vi "Consumer Loop.vi"(8 "error in (no error)":errorcluster) -> (0 "error out":errorcluster)   [LabVIEW 2014]
doc: "Executes the motion commands."
uses:
  Functional_Global/Typedef_Message_Queue_Action.ctl
  Typedef/Typedef_Motor_Message.ctl
  EMC API/EMC_Typedef_Motor_Parameters.ctl
  Typedef/Typedef_Coordinate_Move_Message.ctl
  Globals/Global Stop.vi
panel:
  out "Iterations":i32
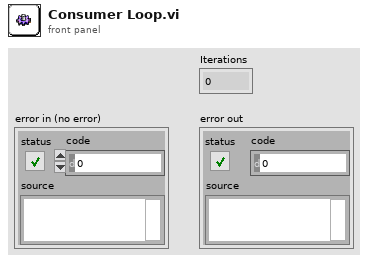
[diagram p1: front panel]
types:
  T1 = typedef "Typedef_Message_Queue_Action.ctl" = enum16{"Init MQueue", "Get MQueue Ref", "Close MQueue"}
  T2 = typedef "Typedef_Motor_Message.ctl" = cluster{"Axis":refnum<k21>, "Motion Parameters":T3}
  T3 = typedef "EMC_Typedef_Motor_Parameters.ctl" = cluster{"position":dbl, "velocity":dbl, "acceleration":dbl, "deceleration":dbl, "accel. jerk":dbl, "decel. jerk":dbl}
  T4 = typedef "Typedef_Coordinate_Move_Message.ctl" = cluster{"position[]":dbl[], "velocity":dbl, "Motion Parameters":T3}
  T5 = typedef "Message Queue.lvlib/Message Cluster.ctl" = cluster{"Message":string, "Message Data":variant}
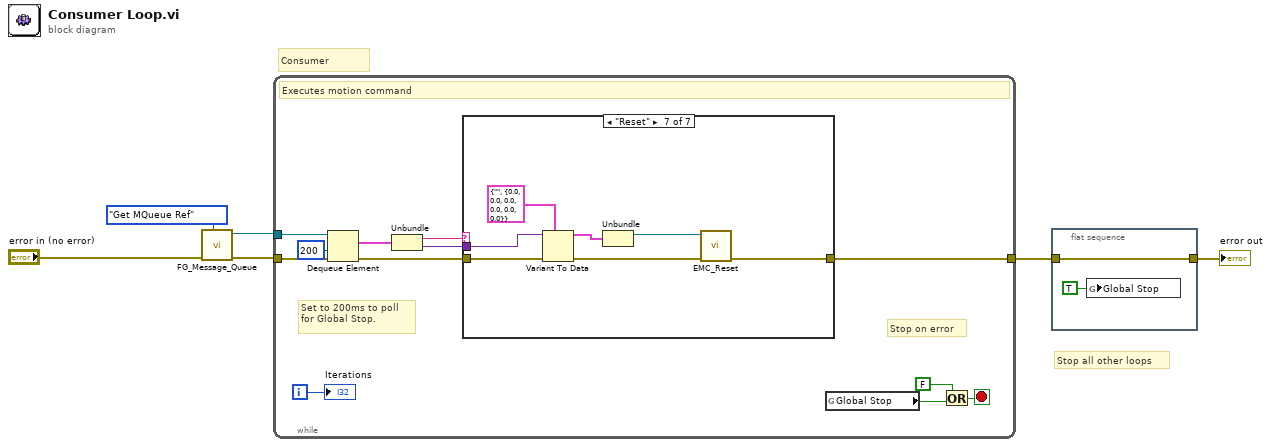
[diagram p0: block diagram]
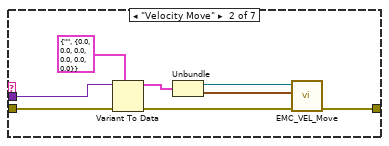
[diagram p3: hidden frame]
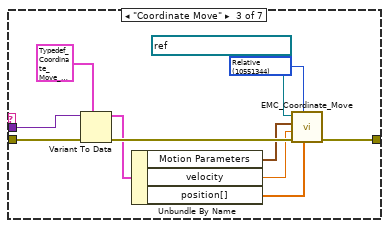
[diagram p4: hidden frame]
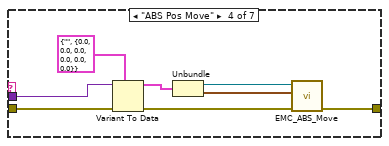
[diagram p5: hidden frame]
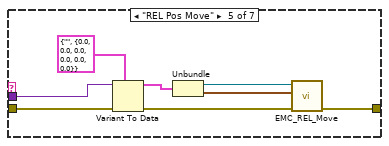
[diagram p6: hidden frame]
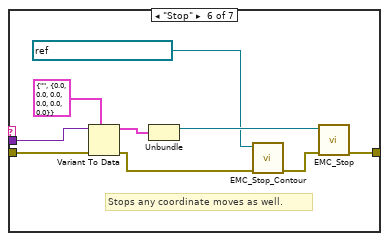
[diagram p7: hidden frame]
diagram:
  # "Stop all other loops"
  # "Consumer"
  n1 = call "FG_Message_Queue.vi"("Action"=Typedef_Message_Queue_Action."Get MQueue Ref", "error in"="error in (no error)") -> ("error out"=w5:errorcluster, "Message Queue"=w4:refnum<queue>)  [unwired: 8 in]
  n2 = while {
    tunnel: w4 -> [w9]
    tunnel: [w11] -> w2
    tunnel: w5 -> [w17]
    i -> [w13]
    stop <- w10 stop-if-true
    # "Stop on error"
    # "Set to 200ms to poll\nfor Global Stop."
    # "Executes motion command"
    n3 = Dequeue Element(queue=w9, timeout in ms (-1)=200, error in (no error)=w17) -> (element=w8:T5, error out=w18:errorcluster)  [unwired: 2 out]
    n4 = Unbundle(w8) -> ("Message"=w16:string, "Message Data"=w15:variant)
    n5 = case shown="\"Reset\"" w16 {
      tunnel: w15 -> [_ w24 w36 w43 w51 w61 w68]
      tunnel: w18 -> [w19 w27 w38 w46 w54 w63 w70]
      tunnel: [w19 w23 w35 w42 w50 w60 w67] -> w11
      frame "Idle", Default {
      }
      frame "Velocity Move" {
        n6 = Variant To Data(error in=w27, type=T2 {"Axis"="", "Motion Parameters"={"position"=0.0, "velocity"=0.0, "acceleration"=0.0, "deceleration"=0.0, "accel. jerk"=0.0, "decel. jerk"=0.0}} ("Motor_Message"), Variant=w24) -> (data=w22:T2, error out=w26:errorcluster)
        n7 = Unbundle(w22) -> ("Axis"=w20:refnum<k21>, "Motion Parameters"=w21:T3)
        n8 = call "EMC_VEL_Move.vi"("error in (no error)"=w26, "Motion Parameters"=w21, "axis"=w20) -> ("error out"=w23:errorcluster)  [unwired: 8 in]
      }
      frame "Coordinate Move" {
        w32 = 10551344 items=["Relative"=10551344, "Absolute"=10551337, "Relative To Capture"=10551345, "Velocity"=10551346, "Polyline"=11600101] ("line move mode")
        n9 = Variant To Data(error in=w38, type=T4 {"position[]"=[], "velocity"=1000.0, "Motion Parameters"={"position"=1000.0, "velocity"=1000.0, "acceleration"=10000.0, "deceleration"=10000.0, "accel. jerk"=10000.0, "decel. jerk"=10000.0}} ("Coordinate_Move_Message"), Variant=w36) -> (data=w31:T4, error out=w37:errorcluster)
        n10 = Unbundle By Name(w31) -> ("Motion Parameters"=w30:T3, "velocity"=w29:dbl, "position[]"=w28:dbl[])
        n11 = call "EMC_Coordinate_Move.vi"("position[]"=w28, "line move mode"=w32, "error in (no error)"=w37, "velocity"=w29, "Motion Parameters"=w30, "resource"=refnum<k21> "Coordinate Space 1") -> ("error out"=w35:errorcluster)  [unwired: 5 in]
      }
      frame "ABS Pos Move" {
        n12 = Variant To Data(error in=w46, type=T2 {"Axis"="", "Motion Parameters"={"position"=0.0, "velocity"=0.0, "acceleration"=0.0, "deceleration"=0.0, "accel. jerk"=0.0, "decel. jerk"=0.0}} ("Motor_Message"), Variant=w43) -> (data=w41:T2, error out=w45:errorcluster)
        n13 = Unbundle(w41) -> ("Axis"=w39:refnum<k21>, "Motion Parameters"=w40:T3)
        n14 = call "EMC_ABS_Move.vi"("error in (no error)"=w45, "Motion Parameters"=w40, "axis"=w39) -> ("error out"=w42:errorcluster)  [unwired: 8 in]
      }
      frame "REL Pos Move" {
        n15 = Variant To Data(error in=w54, type=T2 {"Axis"="", "Motion Parameters"={"position"=0.0, "velocity"=0.0, "acceleration"=0.0, "deceleration"=0.0, "accel. jerk"=0.0, "decel. jerk"=0.0}} ("Motor_Message"), Variant=w51) -> (data=w49:T2, error out=w53:errorcluster)
        n16 = Unbundle(w49) -> ("Axis"=w47:refnum<k21>, "Motion Parameters"=w48:T3)
        n17 = call "EMC_REL_Move.vi"("error in (no error)"=w53, "Motion Parameters"=w48, "axis"=w47) -> ("error out"=w50:errorcluster)  [unwired: 8 in]
      }
      frame "Stop" {
        # "Stops any coordinate moves as well."
        n18 = Variant To Data(error in=w63, type=T2 {"Axis"="", "Motion Parameters"={"position"=0.0, "velocity"=0.0, "acceleration"=0.0, "deceleration"=0.0, "accel. jerk"=0.0, "decel. jerk"=0.0}} ("Motor_Message"), Variant=w61) -> (data=w59:T2, error out=w55:errorcluster)
        n19 = Unbundle(w59) -> ("Axis"=w58:refnum<k21>)  [unwired: 1 out]
        n20 = call "EMC_Stop_Contour.vi"("error in (no error)"=w55, "coordinate"=refnum<k21> "Coordinate Space 1") -> ("error out"=w56:errorcluster)  [unwired: 9 in]
        n21 = call "EMC_Stop.vi"("error in (no error)"=w56, "axis"=w58) -> ("error out"=w60:errorcluster)  [unwired: 8 in, 1 out]
      }
      frame "Reset" {
        n22 = Variant To Data(error in=w70, type=T2 {"Axis"="", "Motion Parameters"={"position"=0.0, "velocity"=0.0, "acceleration"=0.0, "deceleration"=0.0, "accel. jerk"=0.0, "decel. jerk"=0.0}} ("Motor_Message"), Variant=w68) -> (data=w66:T2, error out=w64:errorcluster)
        n23 = Unbundle(w66) -> ("Axis"=w65:refnum<k21>)  [unwired: 1 out]
        n24 = call "EMC_Reset.vi"("error in (no error)"=w64, "axis"=w65) -> ("error out"=w67:errorcluster)  [unwired: 9 in]
      }
    }
    n25 = global read "Global Stop.vi" "Global Stop"() -> (w12:bool)
    n26 = Or(x=FALSE, y=w12) -> (x .or. y?=w10:bool)
    "Iterations" <- w13
  }
  n27 = flat-sequence {
    tunnel: w2 -> [w71]
    tunnel: [w71] -> w1
    frame #0 {
      n28 = global write "Global Stop.vi" "Global Stop"(TRUE ("stop")) -> ()
    }
  }
  "error out" <- w1
